vi "DB_GET TABLE.vi"(11 "MONEY":T2) -> (0 "error out":errorcluster, 1 "Array":string[][](array[string]), 2 "columns":string[](array[string]), 3 "Refnum out":T1)   [LabVIEW 2019, in "CONFIGURATION.lvlib"]
uses:
  Libraries/CONFIGURATION/CONFIGURATION.lvlib
  Libraries/DB_VENDING MACHINE/Type Defs/MONEY.ctl
  <vilib>/addons/database/Connection.llb/Conn ObjectReference.ctl
  <vilib>/addons/database/_DB Variant To Data/Database Variant To Data.xnode
  Libraries/DB_VENDING MACHINE/DB_VENDING MACHINE.lvlib
  <vilib>/addons/database/NI_Database_API.lvlib
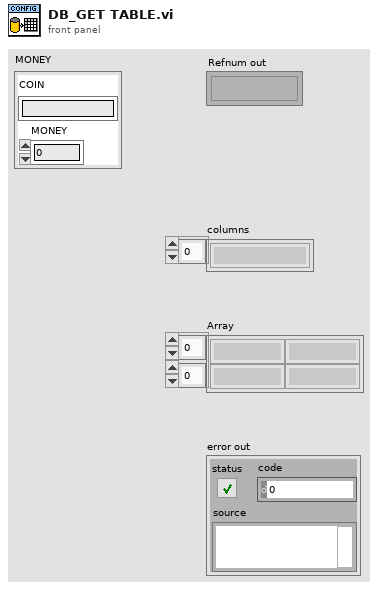
[diagram p1: front panel]
types:
  T1 = typedef "NI_Database_API.lvlib/Conn ObjectReference.ctl" = refnum<k1>
  T2 = typedef "DB_VENDING MACHINE.lvlib/MONEY.ctl" = cluster{"COIN":string, "MONEY":dbl}
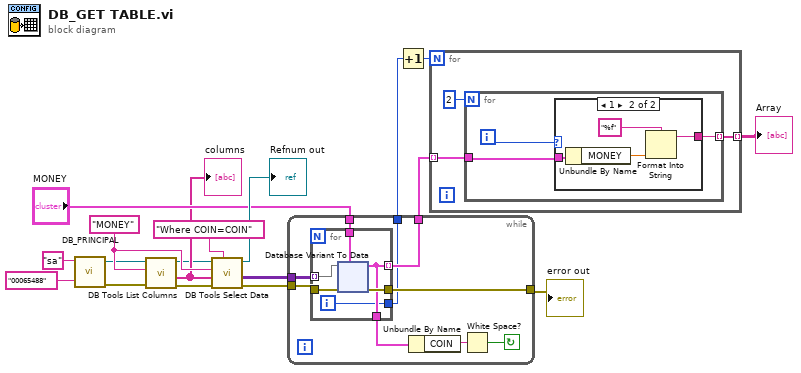
[diagram p0: block diagram]
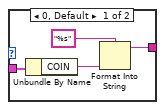
[diagram p2: hidden frame]
diagram:
  w14 = "MONEY" ("table")
  n1 = call "DB_PRINCIPAL.vi"("password"="00065488", "userID"="sa") -> ("error out"=w8:errorcluster, "connection reference"=w7:T1)  [unwired: 8 in]
  n2 = call <vilib>:"DB Tools List Columns.vi"("error in (no error)"=w8, "table"=w14, "connection reference"=w7) -> ("error out"=w12:errorcluster, "columns"=w13:string[], "connection reference out"=w11:T1)  [unwired: 1 in, 1 out]
  "columns" <- w13
  n3 = call <vilib>:"DB Tools Select Data.vi"("condition"="Where COIN=COIN", "error in (no error)"=w12, "columns"=w13, "table"=w14, "connection reference"=w11) -> ("error out"=w5:errorcluster, "data"=w16:variant[][], "connection reference out"=→"Refnum out":T1)  [unwired: 1 in]
  n4 = while {
    tunnel: w16 -> [w27]
    tunnel: w5 -> [w25]
    tunnel: [w24] -> w4
    tunnel: "MONEY" -> [w26]
    tunnel: [w23] -> w3
    tunnel: [w19] -> w2
    stop <- w22 continue-if-true
    n5 = for {
      tunnel: w25 -> [w33]
      tunnel: w26 -> [w32]
      tunnel: w27 -> [w31] mode=indexing
      tunnel: [w29] -> w23 mode=indexing
      tunnel: [w30] -> w24
      tunnel: [w29] -> w20
      tunnel: [w28] -> w19
      i -> [w28]
      n6 = xnode "Database Variant To Data"("database variant"=w31, "error in (no error)"=w33, "type"=w32) -> ("data"=w29:T2, "error out"=w30:errorcluster)
    }
    n7 = Unbundle By Name(w20) -> ("COIN"=w21:string)
    n8 = White Space?(1:w21) -> (0:w22:bool)
  }
  "error out" <- w4
  n9 = Increment(x=w2) -> (x+1=w1:i32)
  n10 = for {
    N: w1 -> [_]
    tunnel: w3 -> [w102] mode=indexing
    tunnel: [w101] -> w6 mode=indexing
    n11 = for {
      N: 2 -> [_]
      tunnel: w102 -> [w105]
      tunnel: [w104] -> w101 mode=indexing
      i -> [w103]
      n12 = case shown="1" w103 {
        tunnel: w105 -> [w109 w113]
        tunnel: [w106 w110] -> w104
        frame 0, Default {
          n13 = Unbundle By Name(w109) -> ("COIN"=w107:string)
          n14 = Format Into String(format string="%s", w107) -> (resulting string=w106:string)  [unwired: 2 in, 1 out]
        }
        frame 1 {
          n15 = Unbundle By Name(w113) -> ("MONEY"=w111:dbl)
          n16 = Format Into String(format string="%f", w111) -> (resulting string=w110:string)  [unwired: 2 in, 1 out]
        }
      }
    }
  }
  "Array" <- w6
